vi "ApplyLanguageToAll.vi"(8 "error in (no error)":errorcluster, 9 "Target Language":string, 10 "Dictionary":T2, 11 "VI Status":T1[](array[typedef])) -> (0 "error out":errorcluster, 3 "VI Status":T1[](array[typedef]))   [LabVIEW 2017, in "JKI Simple Localization.lvlib"]
uses:
  API/JKI Simple Localization.lvlib
  Definitions/Dictionary--Cluster.ctl
  Definitions/Private/Font -- Cluster.ctl
  Definitions/Private/Phrase Dictionary Entry -- Cluster.ctl
  Definitions/Private/VI Info -- Cluster.ctl
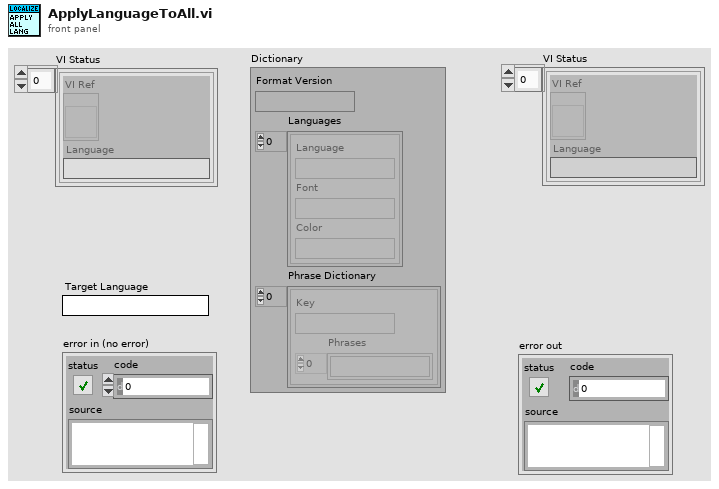
[diagram p1: front panel]
types:
  T1 = typedef "JKI Simple Localization.lvlib/VI Info -- Cluster.ctl" = cluster{"VI Ref":refnum<vi>, "Language":string}
  T2 = typedef "JKI Simple Localization.lvlib/Dictionary--Cluster.ctl" = cluster{"Format Version":string, "Languages":T3[], "Phrase Dictionary":T4[]}
  T3 = typedef "JKI Simple Localization.lvlib/Font -- Cluster.ctl" = cluster{"Language":string, "Font":string, "Color":string}
  T4 = typedef "JKI Simple Localization.lvlib/Phrase Dictionary Entry -- Cluster.ctl" = cluster{"Key":string, "Phrases":string[]}
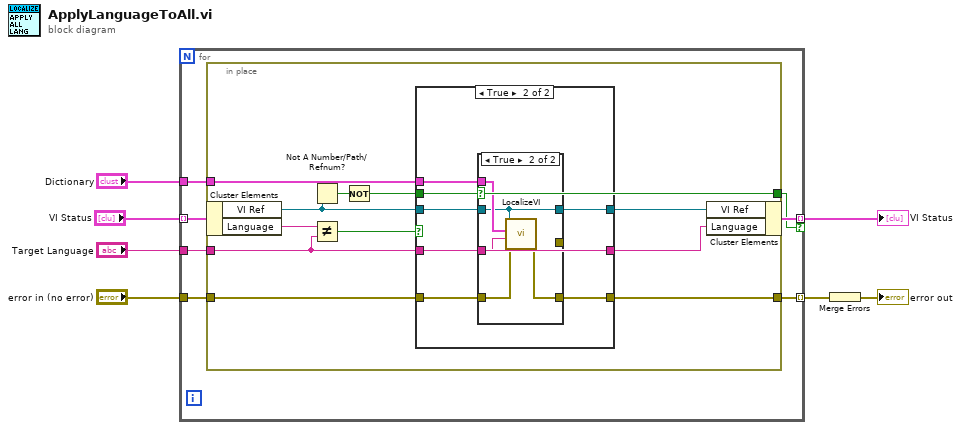
[diagram p0: block diagram]
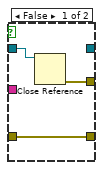
[diagram p3: hidden frame]
diagram:
  n1 = for {
    tunnel: "Dictionary" -> [w12]
    tunnel: "VI Status" -> [w10] mode=indexing
    tunnel: "Target Language" -> [w11]
    tunnel: "error in (no error)" -> [w14]
    tunnel: [w13] -> w4 mode=indexing
    tunnel: [w9] -> w1 mode=indexing if=w8
    n2 = in-place {
      in-place-border: w14 -> [w25]
      in-place-border: [w24] -> w13
      in-place-border: w12 -> [w23]
      in-place-border: w11 -> [w21]
      in-place-border: [w15] -> w8
      n3 = in-place-cluster #1(w10) -> ("VI Ref"=w19:refnum<vi>, "Language"=w18:string)
      n4 = Not A Number/Path/Refnum?(number/path/refnum=w19) -> (NaN/Path/Refnum?=w22:bool)
      n5 = Not Equal?(x=w18, y=w21) -> (x != y?=w20:bool)
      n6 = Not(x=w22) -> (.not. x?=w15:bool)
      n7 = case shown="True" w20 {
        tunnel: w25 -> [w28 w35]
        tunnel: [w28 w34] -> w24
        tunnel: w23 -> [_ w33]
        tunnel: w15 -> [_ w32]
        tunnel: w19 -> [w27 w31]
        tunnel: w21 -> [w26 w30]
        tunnel: [w27 w29] -> w17
        tunnel: [w26 w30] -> w16
        frame False {
        }
        frame True {
          n8 = case shown="True" w32 {
            tunnel: w35 -> [w38 w43]
            tunnel: [w38 w42] -> w34
            tunnel: w33 -> [_ w41]
            tunnel: w30 -> [_ w40]
            tunnel: w31 -> [w37 w39]
            tunnel: [w36 _] -> _
            tunnel: [_ w39] -> w29
            frame False {
              n9 = Close Reference(reference=w37) -> (error out=w36:errorcluster)  [unwired: 1 in]
            }
            frame True {
              n10 = call "LocalizeVI.vi"("error in (no error)"=w43, "Target Language"=w40, "Dictionary"=w41, "VI in"=w39) -> ("error out"=w42:errorcluster)  [unwired: 7 in]
            }
          }
        }
      }
      n11 = in-place-cluster #1("VI Ref"=w17, "Language"=w16) -> (w9:T1)
    }
  }
  "VI Status" <- w1
  n12 = Merge Errors(w4) -> (→"error out":errorcluster)
